vi "Open measure - global.vi"() -> ()   [LabVIEW 2019]
panel:
  in  "Path":path
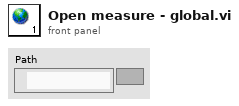
[diagram p1: front panel]
diagram:
